vi "Process Laser State.vi"(7 "error in (no error)":errorcluster, 9 "Data":string, 10 "object in":refnum<class "Laser Ethernet Rack.lvclass">) -> (0 "error out":errorcluster, 3 "object out":refnum<class "Laser Ethernet Rack.lvclass">)   [LabVIEW 2023, in "Laser Ethernet Rack.lvclass"]
uses:
  Laser Ethernet Rack.lvclass
  Laser Ethernet Rack.lvclass/Laser Ethernet Rack.ctl
  <vilib>/Utility/Data Type/NI_Data Type.lvlib
  raw_status.ctl
panel:
  in  "Status":T1
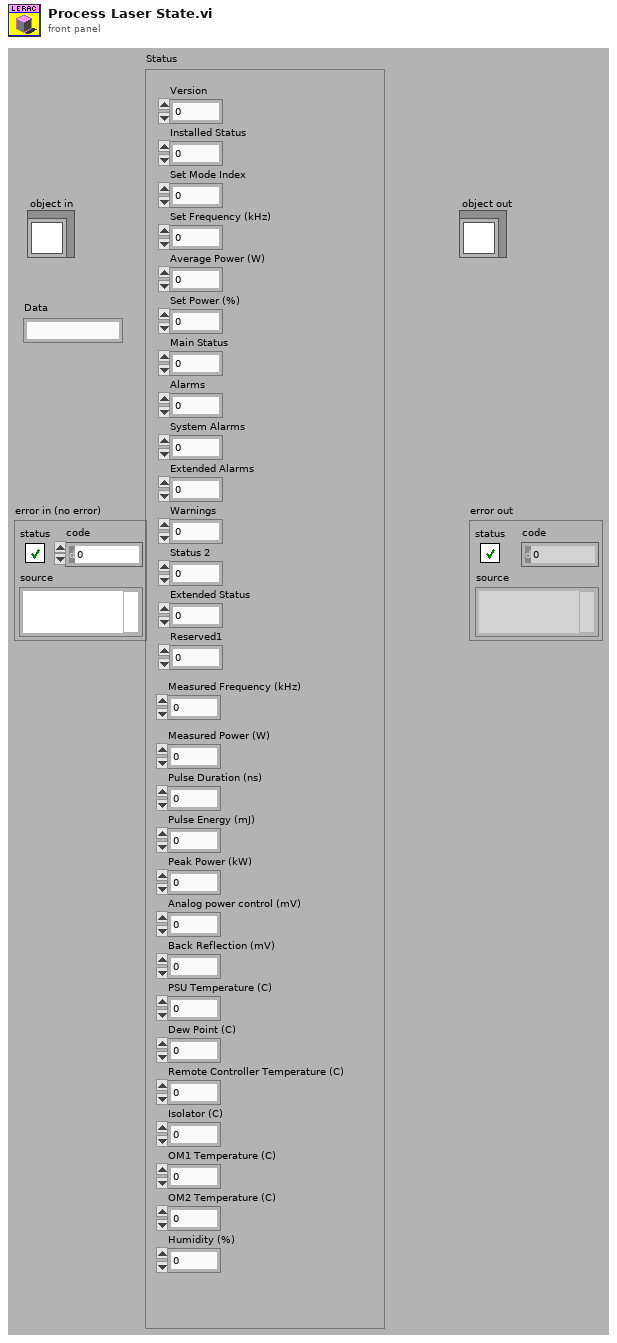
[diagram p1: front panel]
types:
  T1 = typedef "Laser Ethernet Rack.lvclass/raw_status.ctl" = cluster{"Version":u16, "Installed Status":u32, "Set Mode Index":u16, "Set Frequency (kHz)":sgl, "Average Power (W)":sgl, "Set Power (%)":sgl, "Main Status":u32, "Alarms":u32, "System Alarms":u32, "Extended Alarms":u32, "Warnings":u32, "Status 2":u32, "Extended Status":u32, "Reserved1":u16, "Measured Frequency (kHz)":sgl, "Measured Power (W)":sgl, "Pulse Duration (ns)":u32, "Pulse Energy (mJ)":sgl, "Peak Power (kW)":sgl, "Analog power control (mV)":sgl, "Back Reflection (mV)":sgl, "PSU Temperature (C)":sgl, "Dew Point (C)":sgl, "Remote Controller Temperature (C)":sgl, "Isolator (C)":sgl, "OM1 Temperature (C)":sgl, "OM2 Temperature (C)":sgl, "Humidity (%)":sgl}
  T2 = typedef "NI_Data Type.lvlib/Data Type.ctl" = enum8{"Invalid Type", "Void", "I8", "I16", "I32", "I64", "U8", "U16", "U32", "U64", "Single Float", "Double Float", "Extended Float", "Single Complex", "Double Complex", "Extended Complex", "Enum U8", "Enum U16", "Enum U32", "Enum U64", "Single Float With Unit", "Double Float With Unit", "Extended Float With Unit", "Single Complex with Unit", "Double Complex with Unit", "Extended Complex with Unit", "Boolean", "String", "Path", "Picture", "Tag", "Array", "Cluster", "Variant", "LV Variant", "Waveform", "Timestamp", "Digital Waveform", "Digital Data", "ExpressData", "Refnum", "External Data", "VI", "Poly VI", "LabVIEW Class Instance", "Fixed Point", "Set Collection", "Map Collection"}
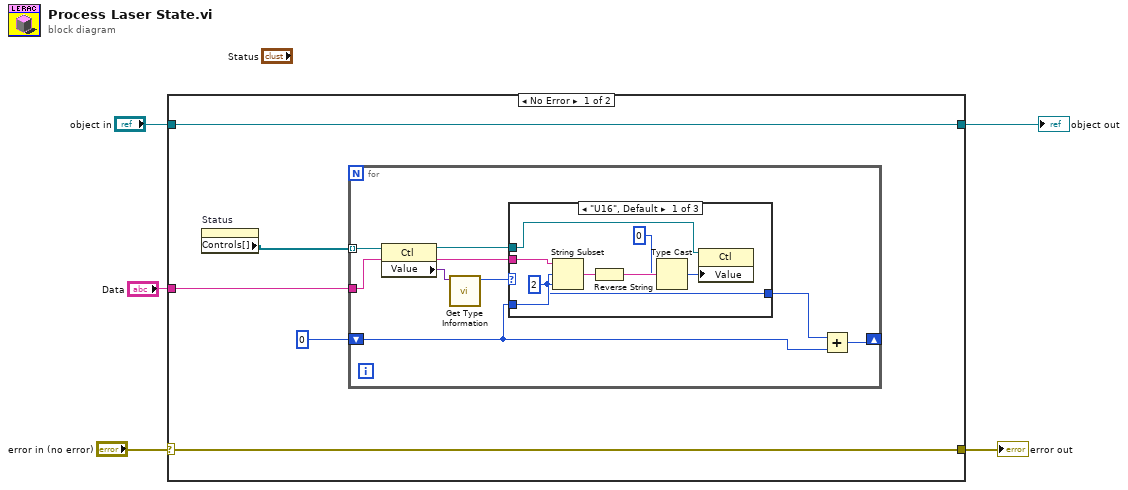
[diagram p0: block diagram]
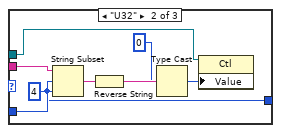
[diagram p2: hidden frame]
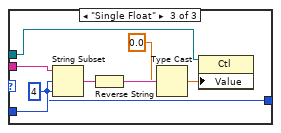
[diagram p3: hidden frame]
diagram:
  n1 = case shown="No Error" "error in (no error)" {
    selector: "error in (no error)" -> [w6 w43]
    tunnel: "Data" -> [w8 _]
    tunnel: "object in" -> [w7 w44]
    tunnel: [w7 w44] -> w2
    tunnel: [w6 w43] -> w1
    frame No Error {
      n2 = property on="Status" class="Clust (strict)"() -> ("Controls[]"=w9:refnum<vi>[])  [unwired: 2 in, 2 out]
      n3 = for {
        tunnel: w9 -> [w15] mode=indexing
        tunnel: w8 -> [w14]
        shift-right: [w11] -> _
        shift-left: 0 ("offset (0)") -> [w12]
        n4 = property class="Ctl"(reference=w15) -> (reference out=w17:refnum<vi>, "Value"=w18:variant)  [unwired: 1 in, 1 out]
        n5 = call <vilib>:"Get Type Information.vi"("variant"=w18) -> ("type"=w16:T2)  [unwired: 6 in, 4 out]
        n6 = case shown="\"U16\", Default" w16 {
          tunnel: w14 -> [w22 w30 w38]
          tunnel: w17 -> [w23 w32 w40]
          tunnel: w12 -> [w20 w28 w36]
          tunnel: [w19 w27 w35] -> w13
          frame "U16", Default {
            w19 = 2
            n7 = String Subset(string=w22, offset (0)=w20, length (rest)=w19) -> (substring=w21:string)
            n8 = Reverse String(1:w21) -> (0:w26:string)
            n9 = Type Cast(type=u16 0, x=w26) -> (*(type *) &x=w24:u16)
            n10 = property class="Ctl"(reference=w23, "Value"=w24) -> ()  [unwired: 1 in, 2 out]
          }
          frame "U32" {
            w27 = 4
            n11 = String Subset(string=w30, offset (0)=w28, length (rest)=w27) -> (substring=w29:string)
            n12 = Reverse String(1:w29) -> (0:w34:string)
            n13 = Type Cast(type=u32 0, x=w34) -> (*(type *) &x=w31:u32)
            n14 = property class="Ctl"(reference=w32, "Value"=w31) -> ()  [unwired: 1 in, 2 out]
          }
          frame "Single Float" {
            w35 = 4
            n15 = String Subset(string=w38, offset (0)=w36, length (rest)=w35) -> (substring=w37:string)
            n16 = Reverse String(1:w37) -> (0:w42:string)
            n17 = Type Cast(type=sgl 0.0, x=w42) -> (*(type *) &x=w39:sgl)
            n18 = property class="Ctl"(reference=w40, "Value"=w39) -> ()  [unwired: 1 in, 2 out]
          }
        }
        n19 = Add(x=w13, y=w12) -> (x+y=w11:i32)
      }
    }
    frame Error {
    }
  }
  "error out" <- w1
  "object out" <- w2
